vi "detect.vi"(2 "rotate\nCCW?":bool) -> (0 "output array":dbl[](array[numeric]), 1 "isSuccess?":bool)   [LabVIEW 2017]
uses:
  <vilib>/myRIO/Instrument Drivers/Utilities/Utilities.lvlib
  <vilib>/myRIO/Common/Instrument Driver Framework/myRIO v1.0/DIO/typedefs/DIO Channels Enum.ctl
  <vilib>/myRIO/Common/Instrument Driver Framework/myRIO v1.0/DIO/typedefs/DIO Channels List.ctl
  <vilib>/myRIO/Common/Instrument Driver Framework/Utilities/typedefs/Generic FPGA Reference.ctl
  <vilib>/myRIO/Common/Instrument Driver Framework/Utilities/typedefs/myRIO v1.0 Reference.ctl
  <vilib>/myRIO/Common/Instrument Driver Framework/Utilities/typedefs/Hardware Version Enum.ctl
  <vilib>/myRIO/Common/Instrument Driver Framework/Utilities/typedefs/myRIO Generic Hardware Reference.ctl
  <vilib>/myRIO/Instrument Drivers/Onboard IO/DIO/typedefs/DIO Reference.ctl
  <vilib>/myRIO/Instrument Drivers/Onboard IO/DIO/DIO.lvlib
  <vilib>/myRIO/Instrument Drivers/Onboard IO/DIO/vis/Write.vi
  <vilib>/myRIO/Instrument Drivers/Onboard IO/DIO/vis/myRIO DIO Open.xnode
  <vilib>/myRIO/Common/Instrument Driver Framework/Utilities/vis/Is FPGA Ref Available.vi
  <vilib>/myRIO/Express VI/Onboard IO/DO/DO Express VI.xnode
  <vilib>/myRIO/Common/Instrument Driver Framework/myRIO v1.0/DIO/vis/myRIO v1.1 Open DIO.vi
  <vilib>/userdefined/High Color/nirio_resource_hc.ctl
panel:
  out "isRotateStop?":bool
  out "Numeric":i32
  in  "degrees I":dbl[](array[numeric])
  in  "detected colors I":string[](array[string])
  out "degree":dbl
  out "thresh":T1(plugin-control)
  out "degrees O":dbl[](array[numeric])
  out "detected colors O":string[](array[string])
  out "isObjectInTheMid":bool
  out "color":string
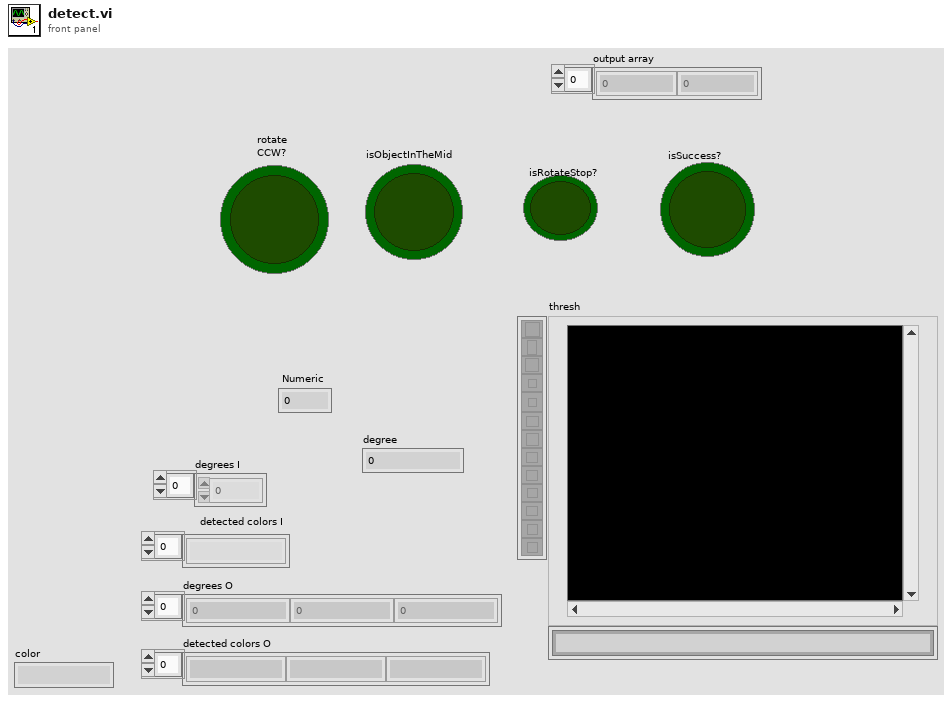
[diagram p1: front panel]
types:
  T1 = typedef "IMAQ Image.ctl" = refnum<image>
  T2 = typedef "DIO.lvlib/DIO Reference.ctl" = cluster{"myRIO Reference":T3, "DIO Channels List":T7}
  T3 = typedef "myRIO Generic Hardware Reference.ctl" = cluster{"myRIO Model":T4, "myRIO Hardware Reference":T5}
  T4 = typedef "Hardware Version Enum.ctl" = enum16{"Unknown", "myRIO-1900", "myRIO-1950", "roboRIO", "NI ELVIS RIO CM"}
  T5 = typedef "myRIO v1.0 Reference.ctl" = cluster{"Generic FPGA Reference":T6, "Allow multiple opens":bool}
  T6 = typedef "Generic FPGA Reference.ctl" = refnum<k20>
  T7 = typedef "DIO Channels List.ctl" = T8[]
  T8 = typedef "DIO Channels Enum.ctl" = enum16{"Not Connected", "C/DIO0", "C/DIO1", "C/DIO2", "C/DIO3", "C/DIO4", "C/DIO5", "C/DIO6", "C/DIO7", "A/DIO0", "A/DIO1", "A/DIO2", "A/DIO3", "A/DIO4", "A/DIO5", "A/DIO6", "A/DIO7", "A/DIO8", "A/DIO9", "A/DIO10", "A/DIO11", "A/DIO12", "A/DIO13", "A/DIO14", "A/DIO15", "B/DIO0", "B/DIO1", "B/DIO2", "B/DIO3", "B/DIO4", "B/DIO5", "B/DIO6", "B/DIO7", "B/DIO8", "B/DIO9", "B/DIO10", "B/DIO11", "B/DIO12", "B/DIO13", "B/DIO14", "B/DIO15", "LED0", "LED1", "LED2", "LED3", "Button0", "DIO/DIO0", "DIO/DIO1", "DIO/DIO2", "DIO/DIO3", "DIO/DIO4", "DIO/DIO5", "DIO/DIO6", "DIO/DIO7", "DIO/DIO8", "DIO/DIO9", "SPI/CS0", "SPI/CS1", "SPI/CS2", "SPI/CS3", "LED RADIO (Green)", "LED RADIO (Red)", "LED COMM (Green)", "LED COMM (Red)", "LED MODE (Green)", "LED MODE (Red)"}
  T9 = typedef "nirio_resource_hc.ctl" = tag
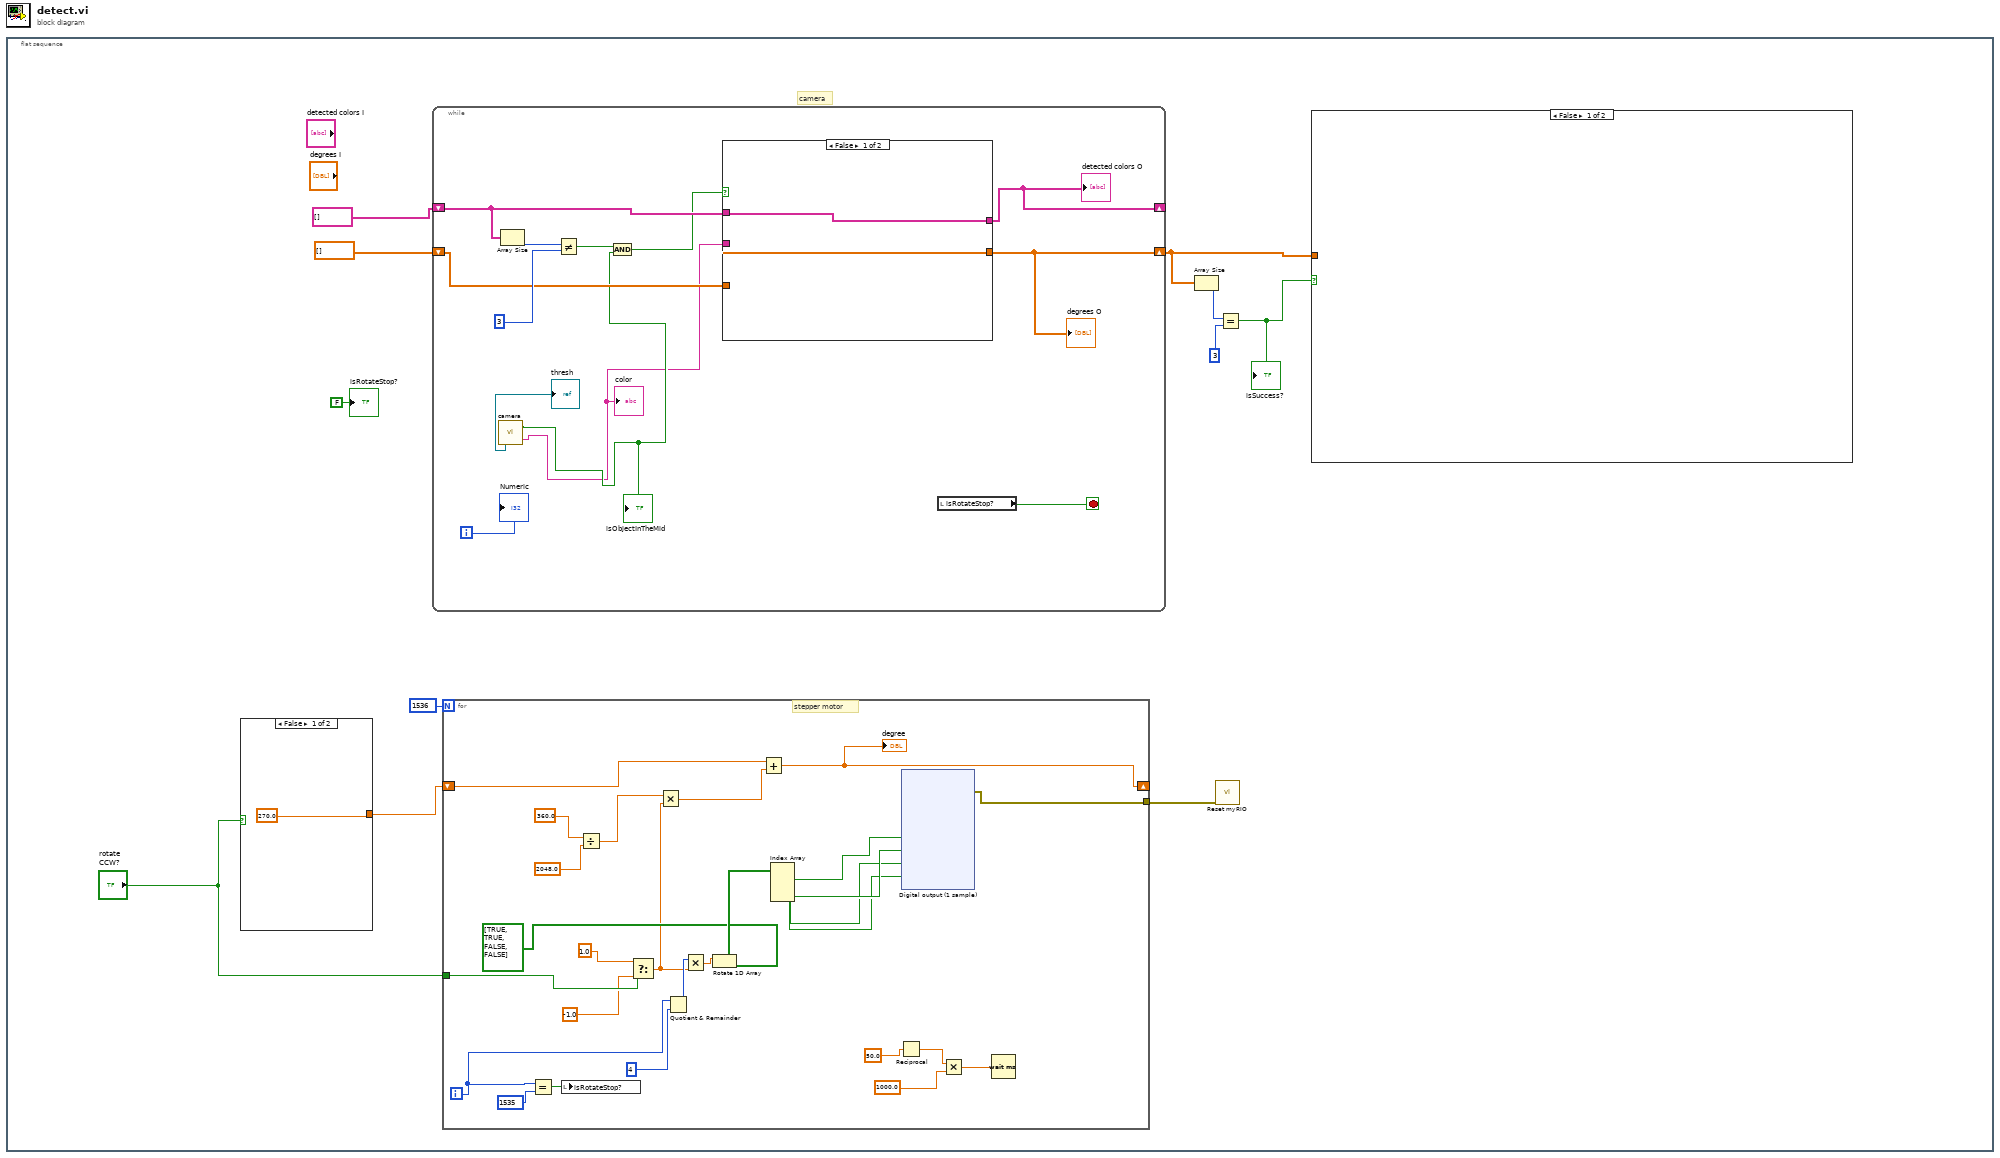
[diagram p0: block diagram]
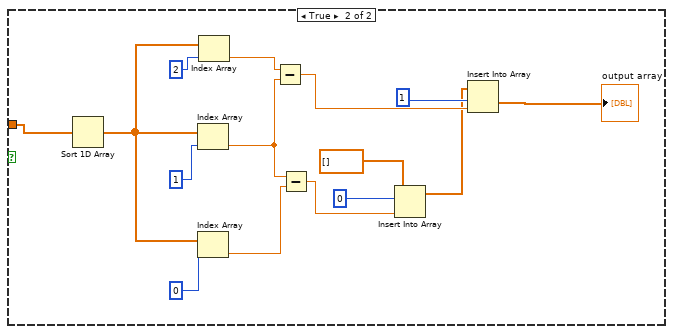
[diagram p2: hidden frame]
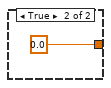
[diagram p3: hidden frame]
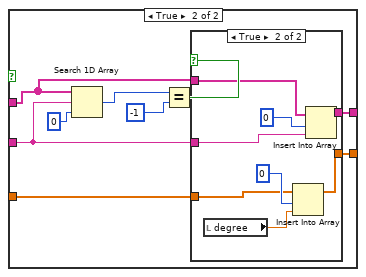
[diagram p4: hidden frame]
diagram:
  n1 = flat-sequence {
    frame #0 {
      # "camera"
      n2 = case shown="False" "rotate\nCCW?" {
        tunnel: [270.0 ("x") 0.0] -> w2
        frame False {
        }
        frame True {
        }
      }
      n3 = while {
        shift-right: [w104] -> _
        shift-left: string[] [] -> [w103]
        shift-right: [w99] -> w8
        shift-left: dbl[] [] -> [w100]
        i -> [w95]
        stop <- w94 stop-if-true
        n4 = call "camera.vi"() -> ("color"=w97:string, "result"=w98:bool, "middle"=→"thresh":T1)  [unwired: 1 in]
        "color" <- w97
        "isObjectInTheMid" <- w98
        n5 = Array Size(array=w103) -> (size(s)=w106:i32)
        n6 = Not Equal?(x=w106, y=3) -> (x != y?=w102:bool)
        n7 = And(x=w102, y=w98) -> (x .and. y?=w101:bool)
        n8 = case shown="False" w101 {
          tunnel: [w108 w117] -> w104
          tunnel: w103 -> [w108 w114]
          tunnel: w97 -> [_ w116]
          tunnel: w100 -> [w107 w110]
          tunnel: [w107 w109] -> w99
          frame False {
          }
          frame True {
            n9 = Search 1D Array(1D array=w114, element=w116, start index (0)=0) -> (index of element=w113:i32)
            n10 = Equal?(x=w113, y=-1) -> (x = y?=w111:bool)
            n11 = case shown="True" w111 {
              tunnel: [w119 w127] -> w117
              tunnel: w116 -> [_ w125]
              tunnel: w114 -> [w119 w124]
              tunnel: w110 -> [w118 w121]
              tunnel: [w118 w122] -> w109
              frame False {
              }
              frame True {
                n12 = local read "degree"() -> (w120:dbl)
                n13 = Insert Into Array(array=w121, index=0, new element=w120) -> (w122:dbl[])
                n14 = Insert Into Array(array=w124, index=0, new element=w125) -> (w127:string[])
              }
            }
          }
        }
        "detected colors O" <- w104
        "degrees O" <- w99
        n15 = local read "isRotateStop?"() -> (w94:bool)
        "Numeric" <- w95
      }
      n16 = for {
        N: 1536 -> [_]
        tunnel: [w53] -> w11
        tunnel: "rotate\nCCW?" -> [w52]
        shift-right: [w37] -> _
        shift-left: w2 -> [w39]
        i -> [w36]
        # "stepper motor"
        n17 = Equal?(x=w36, y=1535) -> (x = y?=w32:bool)
        n18 = local write "isRotateStop?"(w32) -> ()
        n19 = Divide(x=360.0, y=2048.0) -> (x/y=w34:dbl)
        n20 = Select(t=1.0, s=w52, f=-1.0 ("y")) -> (s? t:f=w33:dbl)
        n21 = Multiply(x=w34, y=w33) -> (x*y=w35:dbl)
        n22 = Quotient & Remainder(x=w36, y=4) -> (x-y*floor(x/y)=w42:i32)  [unwired: 1 out]
        n23 = Multiply(x=w42, y=w33) -> (x*y=w43:dbl)
        n24 = Rotate 1D Array(1:bool[] [TRUE, TRUE, FALSE, FALSE], 2:w43) -> (0:w50:bool[])
        n25 = Add(x=w39, y=w35) -> (x+y=w37:dbl)
        "degree" <- w37
        n26 = Index Array(array=w50) -> (element #1=w47:bool, element #2=w46:bool, element #3=w45:bool, element #4=w44:bool)  [unwired: 4 in]
        n27 = Reciprocal(x=50.0 ("milliseconds to wait")) -> (1/x=w29:dbl)
        n28 = xnode "Digital output (1 sample)"("A/DIO0 (Pin 11)"=w47, "A/DIO1 (Pin 13)"=w46, "A/DIO2 (Pin 15)"=w45, "A/DIO3 (Pin 17)"=w44) -> ("error out"=w53:errorcluster)  [unwired: 1 in]
        n29 = Multiply(x=w29, y=1000.0) -> (x*y=w28:dbl)
        n30 = Wait (ms)(milliseconds to wait=w28) -> ()  [unwired: 1 out]
      }
      n31 = Array Size(array=w8) -> (size(s)=w10:i32)
      n32 = call <vilib>:"Reset myRIO.vi"("error in (no error)"=w11) -> ()  [unwired: 10 in, 1 out]
      n33 = Equal?(x=w10, y=3) -> (x = y?=w7:bool)
      "isSuccess?" <- w7
      n34 = case shown="False" w7 {
        tunnel: w8 -> [_ w14]
        frame False {
        }
        frame True {
          n35 = Sort 1D Array(array=w14) -> (sorted array=w23:dbl[])
          n36 = Index Array(array=w23, index=1) -> (element=w24:dbl)
          n37 = Index Array(array=w23, index=0) -> (element=w25:dbl)
          n38 = Index Array(array=w23, index=2) -> (element=w13:dbl)
          n39 = Subtract(x=w13, y=w24) -> (x-y=w21:dbl)
          n40 = Subtract(x=w24, y=w25) -> (x-y=w22:dbl)
          n41 = Insert Into Array(array=dbl[] [], index=0, new element=w22) -> (w12:dbl[])
          n42 = Insert Into Array(array=w12, index=1, new element=w21) -> (→"output array":dbl[])
        }
      }
      "isRotateStop?" <- FALSE ("isRotateStop?")
    }
  }
